vi "CoboltLaser_OutputPowerRead.vi"(0 "ComPort":refnum<visa-resource-name>, 3 "CheckResponse":bool=TRUE, 7 "ErrorIn":errorcluster) -> (20 "ComPortOut":refnum<visa-resource-name>, 21 "OutputPower":dbl format="%.4g", 27 "ErrorOut":errorcluster)   [LabVIEW 2012, in "Cobolt.lvclass"]
doc: "Use this template to build a VI to use as a subVI."
uses:
  Template/Cobolt.lvclass
panel:
  out "ResponseOK":bool
  out "Response":string
  # "(W)"
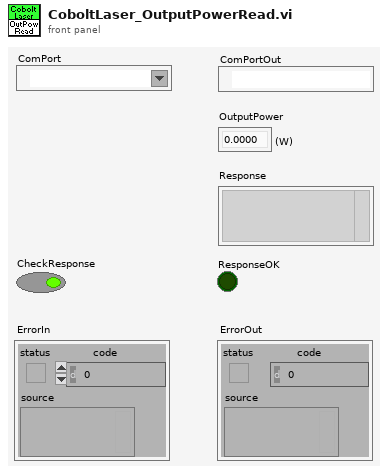
[diagram p1: front panel]
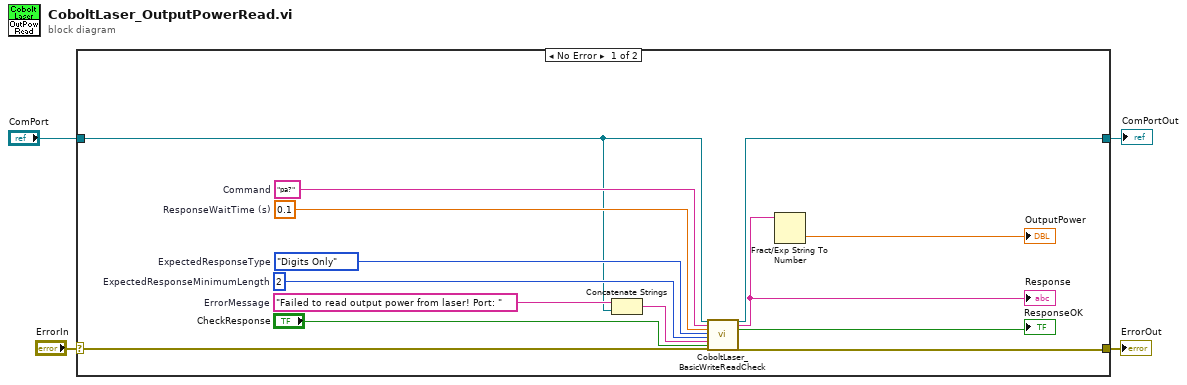
[diagram p0: block diagram]
diagram:
  n1 = case shown="No Error" "ErrorIn" {
    selector: "ErrorIn" -> [w18 w20]
    tunnel: [w17 w20] -> w3
    tunnel: "ComPort" -> [w6 w19]
    tunnel: [w5 w19] -> w1
    frame No Error {
      w13 = 2  # ExpectedResponseMinimumLength
      w14 = enum16{"Any", "Digits Only", "Non-Digits Only"}."Digits Only"  # ExpectedResponseType
      w16 = 0.1  # ResponseWaitTime (s)
      w10 = "Failed to read output power from laser! Port: "  # ErrorMessage
      w15 = "pa?"  # Command
      n2 = Concatenate Strings(w10, w6) -> (w9:string)
      n3 = call "CoboltLaser_BasicWriteReadCheck.vi"("ComPort"=w6, "Command"=w15, "ResponseWaitTime (s)"=w16, "ExpectedResponseType"=w14, "ExpectedResponseMinimumLength"=w13, "ErrorMessage"=w9, "CheckResponse"="CheckResponse", "error in (no error)"=w18) -> ("ComPortOut"=w5:refnum<visa-resource-name>, "Response"=w8:string, "ResponseOK"=→"ResponseOK":bool, "error out"=w17:errorcluster)  [unwired: 16 in]
      "Response" <- w8
      n4 = Fract/Exp String To Number(string=w8) -> (number=→"OutputPower":dbl)  [unwired: 3 in, 1 out]
    }
    frame Error {
    }
  }
  "ErrorOut" <- w3
  "ComPortOut" <- w1
